vi "Icons Location.vi"() -> (2 "Icons Location":path)   [LabVIEW 2020, in "RxnRover.lvlib" / "File IO.lvlib" / "Project Locations.lvlib"]
doc: "Returns the location of default files for the application, independent of whether it is run with the LabVIEW runtime, as a standalone EXE, using an installer, or during development in LabVIEW."
uses:
  Project Locations.lvlib
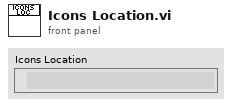
[diagram p1: front panel]
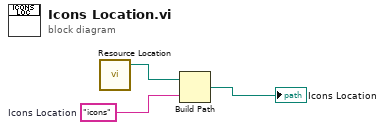
[diagram p0: block diagram]
diagram:
  w3 = "icons"  # Icons Location
  n1 = call "Resource Location.vi"() -> ("Resource Location"=w1:path)  [unwired: 2 in]
  n2 = Build Path(base path=w1, name or relative path=w3) -> (appended path=→"Icons Location":path)
